vi "V_Gain.vi"(1 "Gain":T1) -> (0 "Gain (x)":dbl)   [LabVIEW 2016]
uses:
  typedefs/Gain-Enum.ctl
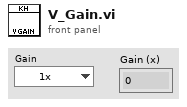
[diagram p1: front panel]
types:
  T1 = typedef "Gain-Enum.ctl" = enum16{"1x", "10x", "100x", "1000x"}
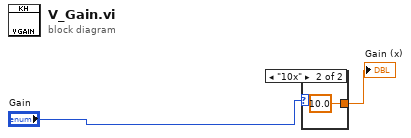
[diagram p0: block diagram]
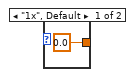
[diagram p2: hidden frame]
diagram:
  n1 = case shown="\"10x\"" "Gain" {
    tunnel: [0.0 ("y") 10.0 ("y")] -> w2
    frame "1x", Default {
    }
    frame "10x" {
    }
  }
  "Gain (x)" <- w2
